vi "Call Msg Send.vi"(7 "Actor":refnum<class "LVCAM.lvclass">, 9 "Priority Msg?":bool, 10 "Msg":refnum<class "Msg.lvclass">) -> (0 "error out":errorcluster)   [LabVIEW 2021, in "LVCAM.lvlib" / "Actor.lvclass"]
uses:
  Actor.lvclass
  Msg/Msg.lvclass
  LVCAM/LVCAM.lvclass
  Actor.lvclass/Actor.ctl
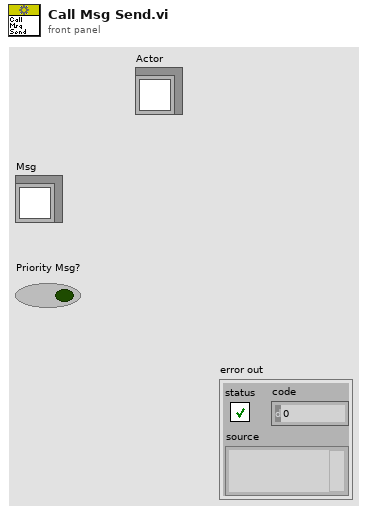
[diagram p1: front panel]
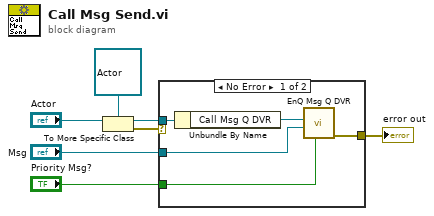
[diagram p0: block diagram]
diagram:
  n1 = To More Specific Class(target class=refnum<class "Actor.lvclass"> refnum ("LVCAM.lvlib:Self Actor.lvclass"), reference="Actor") -> (specific class reference=w3:refnum<class "Actor.lvclass">, error out=w1:errorcluster)  [unwired: 1 in]
  n2 = case shown="No Error" w1 {
    selector: w1 -> [_ w13]
    tunnel: "Msg" -> [w10 _]
    tunnel: [w8 w13] -> w6
    tunnel: "Priority Msg?" -> [w9 _]
    tunnel: w3 -> [w12 _]
    frame No Error {
      n3 = Unbundle By Name(w12) -> ("Call Msg Q DVR"=w11:refnum<data-value>)
      n4 = call "EnQ Msg Q DVR.vi"("Priority Msg?"=w9, "Msg"=w10, "Msg Q DVR"=w11) -> ("error out"=w8:errorcluster)  [unwired: 8 in]
    }
    frame Error {
    }
  }
  "error out" <- w6
